vi "Read Client_Config.vi"(8 "error in (no error)":errorcluster, 11 "Sensor in":refnum<class "Sensor.lvclass">) -> (0 "error out":errorcluster, 2 "Client_Config":T1={"source_ip"="127.0.01", "destination_port"=4370, "detector_calibration"=path "", "detector_configuration"=path ""}, 3 "Sensor out":refnum<class "Sensor.lvclass">)   [LabVIEW 2018, in "Sensor.lvlib" / "Sensor.lvclass"]
uses:
  Sensor.lvclass
  Sensor.lvclass/Sensor.ctl
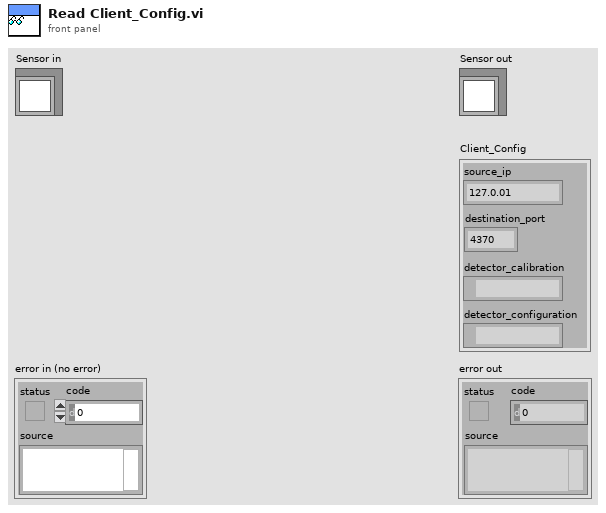
[diagram p1: front panel]
types:
  T1 = cluster{"source_ip":string, "destination_port":u16, "detector_calibration":path, "detector_configuration":path}
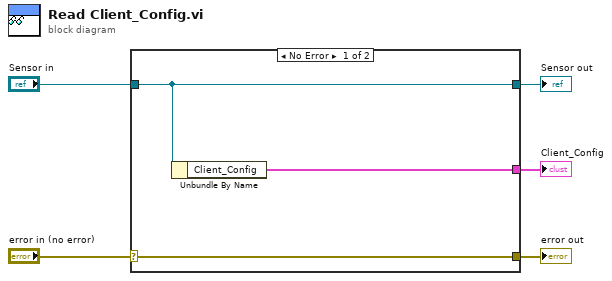
[diagram p0: block diagram]
diagram:
  n1 = case shown="No Error" "error in (no error)" {
    selector: "error in (no error)" -> [w8 w9]
    tunnel: [w8 w9] -> w4
    tunnel: [w7 w10] -> w2
    tunnel: "Sensor in" -> [w7 w10]
    tunnel: [w6 _] -> w1
    frame No Error {
      n2 = Unbundle By Name(w7) -> ("Client_Config"=w6:T1)
    }
    frame Error {
    }
  }
  "error out" <- w4
  "Sensor out" <- w2
  "Client_Config" <- w1
